vi "create_image_subselection.vi"(6 "Animal x":i32, 8 "Full image":i32[][](array[numeric])) -> (0 "Animal x\nimage subselection":i32[][](array[numeric]))   [LabVIEW 2011]
uses:
  Action Items.ctl
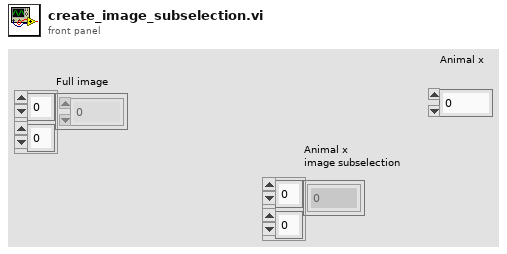
[diagram p1: front panel]
types:
  T1 = typedef "Action Items.ctl" = enum16{"Initialize", "Get"}
  T2 = cluster{"# X-pixel per animal":i32, "# Y-pixel per animal":i32, "Start x-pixel of animals":i32[], "Start y-pixel of animals":i32[]}
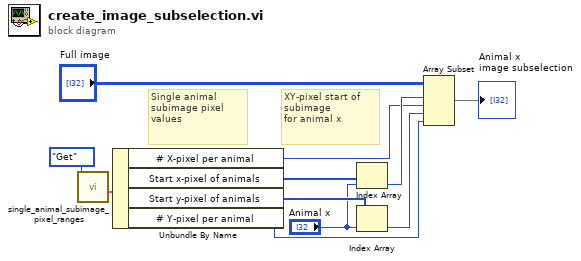
[diagram p0: block diagram]
diagram:
  # "XY-pixel start of subimage \nfor animal x"
  # "Single animal \nsubimage pixel\nvalues"
  n1 = call "single_animal_subimage_pixel_ranges.vi"("Action"=Action_Items."Get") -> ("Single animal\nsubimage pixel\nranges"=w3:T2)  [unwired: 10 in]
  n2 = Unbundle By Name(w3) -> ("# X-pixel per animal"=w2:i32, "Start x-pixel of animals"=w1:i32[], "Start y-pixel of animals"=w11:i32[], "# Y-pixel per animal"=w10:i32)
  n3 = Index Array(array=w1, index="Animal x") -> (element=w8:i32)
  n4 = Index Array(array=w11, index="Animal x") -> (element=w9:i32)
  n5 = Array Subset(array="Full image", index (row)=w8, length (row)=w2, index (col)=w9, length (col)=w10) -> (→"Animal x\nimage subselection":i32[][])
